vi "Get ID from name.vi"(8 "error in (no error)":errorcluster, 11 "Name":string) -> (0 "error out":errorcluster, 1 "found?":bool, 3 "id out":i32)   [LabVIEW 2020, in "MCP Server.lvlib"]
uses:
  MCP Server.lvlib
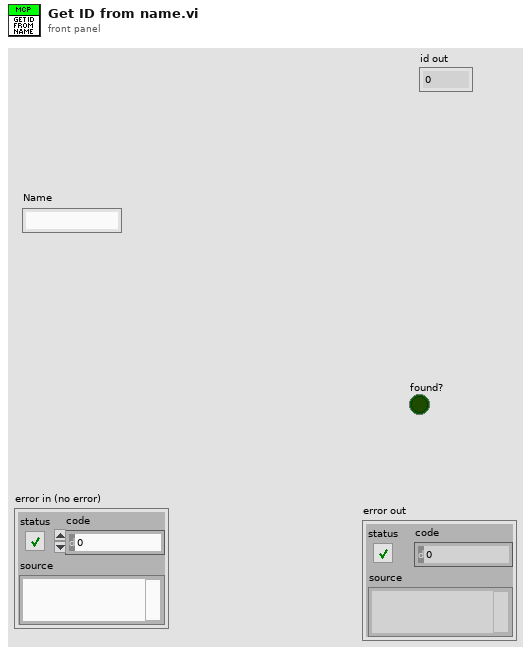
[diagram p1: front panel]
types:
  T1 = enum16{"Get", "GetAll", "Add", "Remove", "Clear"}
  T2 = typedef "MCP Server.lvlib/Server Data.ctl" = cluster{"Name":string, "Description":string, "Tools":T3[], "Parameters":string[][], "Logging Info":T6, "User Events":T7, "Prompts":T8[], "resources":T10[], "HTTP Server":refnum<class "Server.lvclass">}
  T3 = typedef "MCP Server.lvlib/Tool Data.ctl" = cluster{"Name":string, "Description":string, "Ignored":string[], "inputs":T4[], "outputs":T5[], "VI Refnum":refnum<vi>}
  T4 = typedef "MCP Server.lvlib/Input Parameter.ctl" = cluster{"name":string, "type":string, "description":string, "required":bool, "raw name":string}
  T5 = typedef "MCP Server.lvlib/Output Parameter.ctl" = cluster{"name":string, "description":string, "type":string, "raw name":string}
  T6 = typedef "MCP Server.lvlib/Logging.ctl" = cluster{"Log":string[], "Max Length":i32}
  T7 = typedef "MCP Server.lvlib/User Events.ctl" = cluster{"onError":refnum<user-event>, "onRpc":refnum<user-event>}
  T8 = typedef "MCP Server.lvlib/Prompt Data.ctl" = cluster{"name":string, "description":string, "arguments":T9[], "return terminal name":string, "results description":string, "VI Refnum":refnum<vi>}
  T9 = typedef "MCP Server.lvlib/Prompt Argument.ctl" = cluster{"name":string, "description":string, "required":bool, "raw_name":string}
  T10 = typedef "MCP Server.lvlib/resource data.ctl" = cluster{"uri":string, "name":string, "description":string, "mimeType":string, "file path":path}
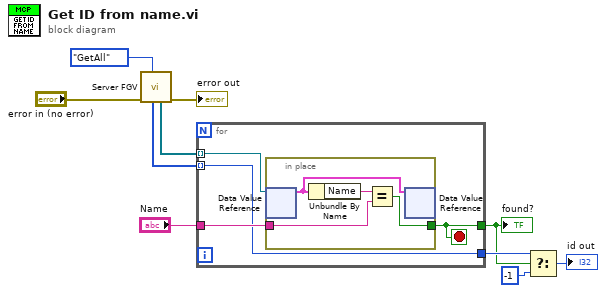
[diagram p0: block diagram]
diagram:
  n1 = call "Server FGV.vi"("Mode"=T1."GetAll", "error in"="error in (no error)") -> ("error out"=→"error out":errorcluster, "all servers"=w6:refnum<data-value>[], "server ids"=w5:i32[])  [unwired: 5 in, 2 out]
  n2 = for {
    tunnel: "Name" -> [w14]
    tunnel: w6 -> [w13] mode=indexing
    tunnel: [w12] -> w2
    tunnel: w5 -> [w11] mode=indexing
    tunnel: [w11] -> w4
    stop <- w12 stop-if-true
    n3 = in-place {
      in-place-border: w14 -> [w16]
      in-place-border: [w15] -> w12
      n4 = in-place-dvr #1(w13) -> (w18:T2)  [unwired: 1 out]
      n5 = Unbundle By Name(w18) -> ("Name"=w17:string)
      n6 = Equal?(x=w17, y=w16) -> (x = y?=w15:bool)
      n7 = in-place-dvr #1(w18) -> ()  [unwired: 2 out]
    }
  }
  "found?" <- w2
  n8 = Select(t=w4, s=w2, f=-1) -> (s? t:f=→"id out":i32)
